vi "Project_Get Build Destination.vi"(8 "error in(no error)":errorcluster, 9 "Target Name(\"\"> My Computer)":string, 10 "Build Specification Name":string, 11 "Project Path":path) -> (0 "error out":errorcluster, 1 "Success?":bool, 3 "Build Destination":path)   [LabVIEW 2019, in "ProjectBuilder.lvlib"]
doc: "Get the build destination from a project for a build specification."
uses:
  ProjectBuilder.lvlib
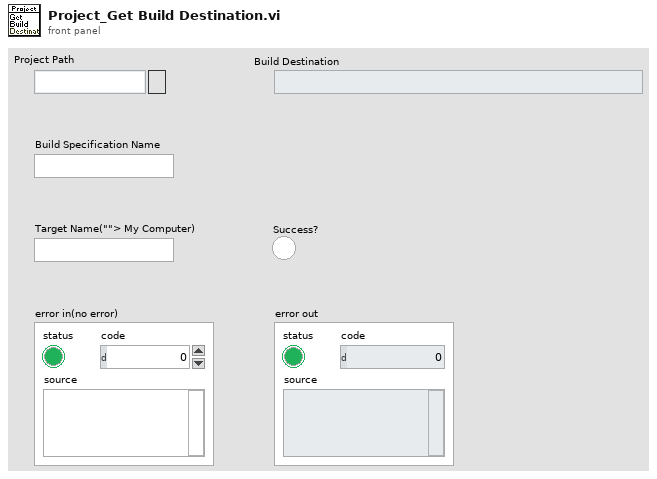
[diagram p1: front panel]
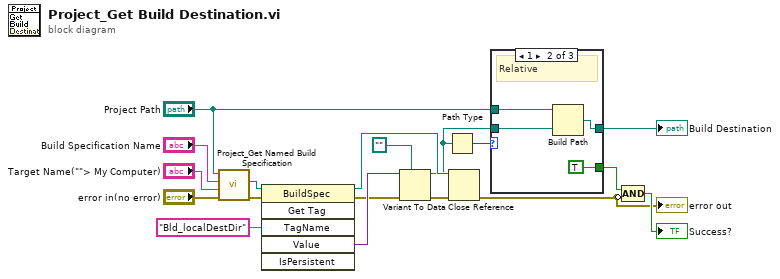
[diagram p0: block diagram]
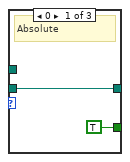
[diagram p2: hidden frame]
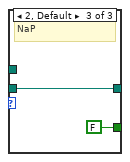
[diagram p3: hidden frame]
diagram:
  n1 = call "Project_Get Named Build Specification.vi"("error in(no error)"="error in(no error)", "Target Name(\"\"> My Computer)"="Target Name(\"\"> My Computer)", "Build Specification Name"="Build Specification Name", "Project Path"="Project Path") -> ("error out"=w16:errorcluster, "Build Spec reference"=w5:refnum<vi>)  [unwired: 4 in, 2 out]
  n2 = invoke class="BuildSpec" method="Get Tag"(reference=w5, error in=w16, "TagName"="Bld_localDestDir") -> (reference out=w18:refnum<vi>, error out=w13:errorcluster, "Value"=w15:variant)  [unwired: 3 in, 3 out]
  n3 = Variant To Data(error in=w13, type=path "", Variant=w15) -> (data=w10:path, error out=w12:errorcluster)
  n4 = Path Type(1:w10) -> (0:w11:i16)
  n5 = Close Reference(reference=w18, error in (no error)=w12) -> (error out=w1:errorcluster)
  "error out" <- w1
  n6 = case shown="1" w11 {
    tunnel: w10 -> [w20 w24 w26]
    tunnel: [w20 w23 w26] -> w4
    tunnel: "Project Path" -> [_ w21 _]
    tunnel: [TRUE TRUE FALSE] -> w3
    frame 0 {
      # "Absolute"
    }
    frame 1 {
      # "Relative"
      n7 = Build Path(base path=w21, name or relative path=w24) -> (appended path=w23:path)
    }
    frame 2, Default {
      # "NaP"
    }
  }
  "Build Destination" <- w4
  n8 = Compound Arithmetic op=AND(w3, invert w1) -> (→"Success?":bool)
